vi "DQMH Show Diagram.vi"(7 "Module Disk Path":path, 8 "error in (no error)":errorcluster, 11 "Application reference":refnum<vi>) -> (0 "error out":errorcluster)   [LabVIEW 2022 SP3, in "hse-dqmh-dynamicrequesters.lvlib"]
doc: "Calls the \"Request UI Display\" request VI of the module in <b>Path to module directory</b>. Hands over the <b>Module Name</b> and the <b>Display Scenario</b>.\n\n____\nHAMPEL SOFTWARE ENGINEERING v3.8.0 (2023-12-18 14:41)"
uses:
  hse-dqmh-dynamicrequesters.lvlib
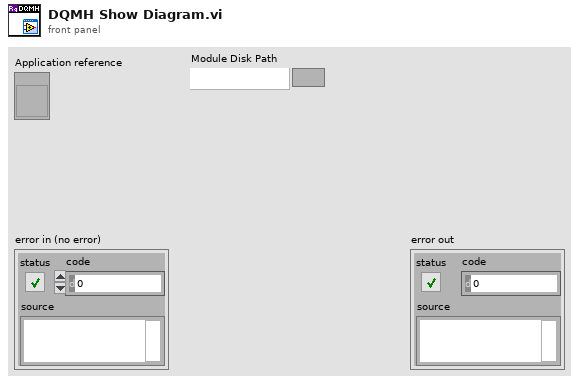
[diagram p1: front panel]
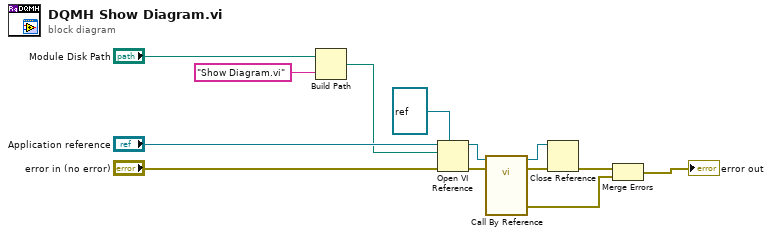
[diagram p0: block diagram]
diagram:
  n1 = Build Path(base path="Module Disk Path", name or relative path="Show Diagram.vi") -> (appended path=w11:path)
  n2 = Open VI Reference(type specifier VI Refnum (for type only)=refnum<vi> refnum, application reference (local)="Application reference", vi path=w11, error in (no error)="error in (no error)") -> (vi reference=w10:refnum<vi>, error out=w9:errorcluster)  [unwired: 2 in]
  n3 = call-by-ref "?"(reference=w10, error in=w9) -> (reference out=w6:refnum<vi>, error out=w7:errorcluster, 0:"error out"=w5:errorcluster)  [unwired: 11 in]
  n4 = Close Reference(reference=w6, error in (no error)=w7) -> (error out=w8:errorcluster)
  n5 = Merge Errors(w8, w5) -> (→"error out":errorcluster)
